vi "DCA Convert 1.2 to 1.8.vi"(1 "DCA 1.2 Test Parameters":T2={"Tag"="", "Use Instrument"=FALSE, "Quick Mode"=FALSE, "Topology"=enum."Pi", "Zo"=50.0, "Range"=0, "Resolution"=0, "Blank Screen"=FALSE, "Limits"=[], "Reports"={"Reports to Generate"=[], "Print Reports"=TRUE}, "Lock Topology"=FALSE} {"Resolution" items=["Auto", "4 1/2", "5 1/2", "6 1/2"]; "Range" items=["Auto", "Min", "Max", "100", "1,000", "10,000", "100,000", "1,000,000", "10,000,000", "100,000,000"]}) -> (0 "DCA 1.8 Test Parameters":T1={"Tag"="", "Use Instrument"=FALSE, "Quick Mode"=FALSE, "Topology"=enum."Pi", "Zo"=50.0, "Range"=0, "Resolution"=0, "Blank Screen"=FALSE, "Limits"=[], "Datasheets"={"Datasheets to Generate"=[], "Print Datasheets"=TRUE}, "Lock Topology"=FALSE, "Normalize"=TRUE, "ATTN Calc"=enum."Power"} {"Resolution" items=["Auto", "4 1/2", "5 1/2", "6 1/2"]; "Range" items=["Auto", "Min", "Max", "100", "1,000", "10,000", "100,000", "1,000,000", "10,000,000", "100,000,000"]; "Limits"."Run" min=1 step=1})   [LabVIEW 2011]
uses:
  TypeDefs/DCA Test Parameters v1.2.ctl
  TypeDefs/DCA Test Parameters v1.8.ctl
panel:
  # "="
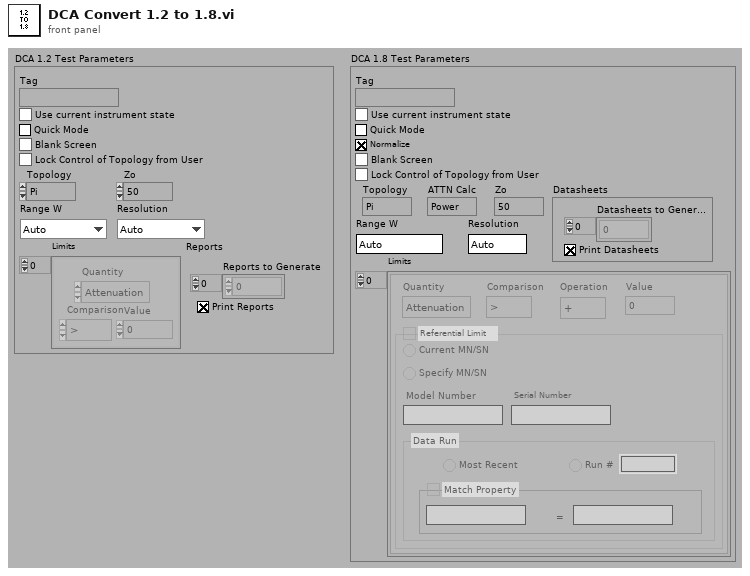
[diagram p1: front panel]
types:
  T1 = typedef "DCA Test Parameters v1.8.ctl" = cluster{"Tag":string, "Use Instrument":bool, "Quick Mode":bool, "Topology":enum32{"Pi", "T"}, "Zo":dbl, "Range":u16, "Resolution":u16, "Blank Screen":bool, "Limits":cluster{"Quantity":enum16{"Attenuation", "Zin", "Zout", "R1", "R2", "R3", "Rab", "Rac", "Rbc"}, "Comparison":enum16{">", ">=", "<", "<=", "+", "-"}, "Operation":enum16{"+", "-"}, "Value":dbl, "Ref Limit":bool, "Ref Type":enum32{"Current", "Specify"}, "Model":string, "Serial":string, "Run Type":enum32{"Most Recent", "Run #"}, "Run":i32, "Match Property":bool, "Property":string, "Property Value":string}[], "Datasheets":cluster{"Datasheets to Generate":i32[], "Print Datasheets":bool}, "Lock Topology":bool, "Normalize":bool, "ATTN Calc":enum32{"Power", "Voltage"}}
  T2 = typedef "DCA Test Parameters v1.2.ctl" = cluster{"Tag":string, "Use Instrument":bool, "Quick Mode":bool, "Topology":enum32{"Pi", "T"}, "Zo":dbl, "Range":u16, "Resolution":u16, "Blank Screen":bool, "Limits":cluster{"Quantity":enum16{"Attenuation", "Zin", "Zout", "R1", "R2", "R3", "Rab", "Rac", "Rbc"}, "Comparison":enum16{">", ">=", "<", "<="}, "Value":dbl}[], "Reports":cluster{"Reports to Generate":i32[], "Print Reports":bool}, "Lock Topology":bool}
  T3 = cluster{"Quantity":enum16{"Attenuation", "Zin", "Zout", "R1", "R2", "R3", "Rab", "Rac", "Rbc"}, "Comparison":enum16{">", ">=", "<", "<=", "+", "-"}, "Operation":enum16{"+", "-"}, "Value":dbl, "Ref Limit":bool, "Ref Type":enum32{"Current", "Specify"}, "Model":string, "Serial":string, "Run Type":enum32{"Most Recent", "Run #"}, "Run":i32, "Match Property":bool, "Property":string, "Property Value":string}[]
  T4 = cluster{"Reports to Generate":i32[], "Print Reports":bool}
  T5 = cluster{"Quantity":enum16{"Attenuation", "Zin", "Zout", "R1", "R2", "R3", "Rab", "Rac", "Rbc"}, "Comparison":enum16{">", ">=", "<", "<="}, "Value":dbl}[]
  T6 = cluster{"Quantity":enum16{"Attenuation", "Zin", "Zout", "R1", "R2", "R3", "Rab", "Rac", "Rbc"}, "Comparison":enum16{">", ">=", "<", "<=", "+", "-"}, "Operation":enum16{"+", "-"}, "Value":dbl, "Ref Limit":bool, "Ref Type":enum32{"Current", "Specify"}, "Model":string, "Serial":string, "Run Type":enum32{"Most Recent", "Run #"}, "Run":i32, "Match Property":bool, "Property":string, "Property Value":string}
  T7 = enum16{"Attenuation", "Zin", "Zout", "R1", "R2", "R3", "Rab", "Rac", "Rbc"}
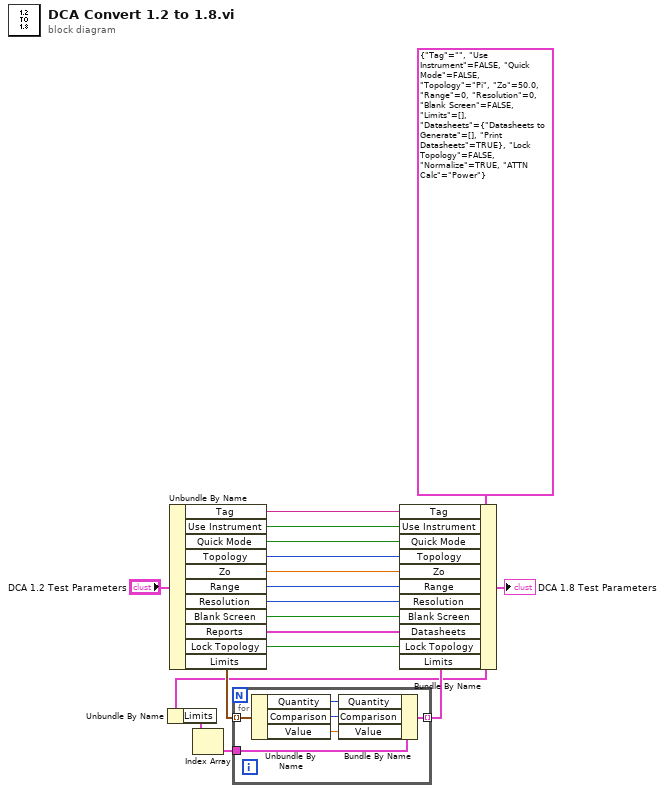
[diagram p0: block diagram]
diagram:
  w1 = T1 {"Tag"="", "Use Instrument"=FALSE, "Quick Mode"=FALSE, "Topology"=enum."Pi", "Zo"=50.0, "Range"=0, "Resolution"=0, "Blank Screen"=FALSE, "Limits"=[], "Datasheets"={"Datasheets to Generate"=[], "Print Datasheets"=TRUE}, "Lock Topology"=FALSE, "Normalize"=TRUE, "ATTN Calc"=enum."Power"} ("DCA 1.9 Test Parameters")
  n1 = Unbundle By Name(w1) -> ("Limits"=w7:T3)
  n2 = Unbundle By Name("DCA 1.2 Test Parameters") -> ("Tag"=w17:string, "Use Instrument"=w16:bool, "Quick Mode"=w15:bool, "Topology"=w14:enum32{"Pi", "T"}, "Zo"=w13:dbl, "Range"=w12:u16, "Resolution"=w11:u16, "Blank Screen"=w10:bool, "Reports"=w9:T4, "Lock Topology"=w8:bool, "Limits"=w5:T5)
  n3 = Index Array(array=w7) -> (element=w6:T6)  [unwired: 1 in]
  n4 = for {
    tunnel: w5 -> [w23] mode=indexing
    tunnel: w6 -> [w22]
    tunnel: [w18] -> w4 mode=indexing
    n5 = Unbundle By Name(w23) -> ("Quantity"=w19:T7, "Comparison"=w20:enum16{">", ">=", "<", "<="}, "Value"=w21:dbl)
    n6 = Bundle By Name(cluster=w22, "Quantity"=w19, "Comparison"=w20, "Value"=w21) -> (w18:T6)
  }
  n7 = Bundle By Name(cluster=w1, "Tag"=w17, "Use Instrument"=w16, "Quick Mode"=w15, "Topology"=w14, "Zo"=w13, "Range"=w12, "Resolution"=w11, "Blank Screen"=w10, "Datasheets"=w9, "Lock Topology"=w8, "Limits"=w4) -> (→"DCA 1.8 Test Parameters":T1)
